vi "Override Error.vi"(10 "Error":errorcluster, 11 "Base Queue in":refnum<class "Base Queue.lvclass">) -> (3 "Base Queue out":refnum<class "Base Queue.lvclass">)   [LabVIEW 2021, in "jettl.lvlib" / "Base Queue.lvlib" / "Base Queue.lvclass"]
uses:
  Base Queue.lvclass
  Base Queue.lvclass/Base Queue.ctl
  State/Error State/Error State.lvclass
  C:/git/jettl/jettl/jettl/Base Queue/State/State/State.lvclass
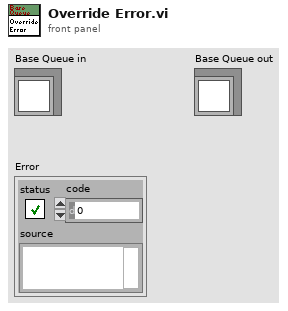
[diagram p1: front panel]
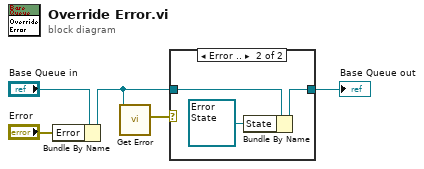
[diagram p0: block diagram]
diagram:
  n1 = Bundle By Name(cluster="Base Queue in", "Error"="Error") -> (w2:refnum<class "Base Queue.lvclass">)
  n2 = call-dynamic "Get Error.vi"("Base Queue in"=w2) -> ("Error"=w3:errorcluster)  [unwired: 10 in]
  n3 = case shown="Error .." w3 {
    tunnel: [w6 w8] -> w1
    tunnel: w2 -> [w6 w9]
    frame No Error {
    }
    frame Error {
      n4 = Bundle By Name(cluster=w9, "State"=refnum<class "Error State.lvclass"> refnum ("jettl.lvlib:jettl Queue Actor.lvlib:Error State.lvclass")) -> (w8:refnum<class "Base Queue.lvclass">)
    }
  }
  "Base Queue out" <- w1
